vi "VI Tree.vi"   [LabVIEW 2021, in "IBM4.lvlib"]
doc: "This is the instrument driver for the <INSTRUMENT NAME>. The VI Tree displays all the user-callable VIs of the instrument driver in an organized table."
uses:
  <instrlib>/IBM4/IBM4.lvlib
panel:
  # "(c) 2014 <Enter Company Name Here>.  ALL RIGHTS RESERVED."
  # "SEE DIAGRAM\nFOR VI TREE."
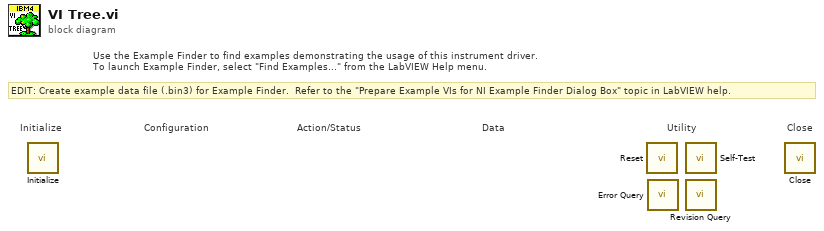
[diagram p0: block diagram]
diagram:
  # "EDIT: Create example data file (.bin3) for Example Finder.  Refer to the \"Prepare Example VIs for NI Example Finder Dialog Box\" topic in LabVIEW help."
  # "Use the Example Finder to find examples demonstrating the usage of this instrument driver.\nTo launch Example Finder, select \"Find Examples...\" from the LabVIEW Help menu."
  # "Configuration"
  # "Utility"
  # "Data"
  # "Action/Status"
  # "Close"
  # "Initialize"
  n1 = call <instrlib>:"Initialize.vi"() -> ()  [unwired: 10 in, 2 out]
  n2 = call <instrlib>:"Reset.vi"() -> ()  [unwired: 10 in, 2 out]
  n3 = call <instrlib>:"Error Query.vi"() -> ()  [unwired: 8 in, 4 out]
  n4 = call <instrlib>:"Self-Test.vi"() -> ()  [unwired: 8 in, 4 out]
  n5 = call <instrlib>:"Revision Query.vi"() -> ()  [unwired: 8 in, 4 out]
  n6 = call <instrlib>:"Close.vi"() -> ()  [unwired: 11 in, 1 out]
